vi "DescribeTextField.vi"(0 "XRef":T15, 1 "ID":T3, 2 "State In":T14) -> (14 "Text Field Info":T2, 15 "Fatal Error Out":T1)   [LabVIEW 2022 SP3, in "Flex Block.xnode"]
uses:
  Flex Block.xnode
  <vilib>/XNodeSupport/XNodeXNodeRef.ctl
  <vilib>/XNodeSupport/XNodeString.ctl
  State.ctl
  <vilib>/XNodeSupport/XNodeTextFieldInfo.ctl
  <vilib>/XNodeSupport/XNodeRect32.ctl
  <vilib>/XNodeSupport/XNodeInt.ctl
  <vilib>/XNodeSupport/XNodeJustification.ctl
  <vilib>/XNodeSupport/XNodeHorizontal.ctl
  <vilib>/XNodeSupport/XNodeVertical.ctl
  <vilib>/XNodeSupport/XNodeColor.ctl
  <vilib>/XNodeSupport/XNodeFont.ctl
  <vilib>/XNodeSupport/XNodeUserFont.ctl
  <vilib>/XNodeSupport/XNodeUInt.ctl
  <vilib>/XNodeSupport/XNodeBool.ctl
  <vilib>/XNodeSupport/XNodeErrorCluster.ctl
  <vilib>/XNodeSupport/NI_XNodeSupport.lvlib
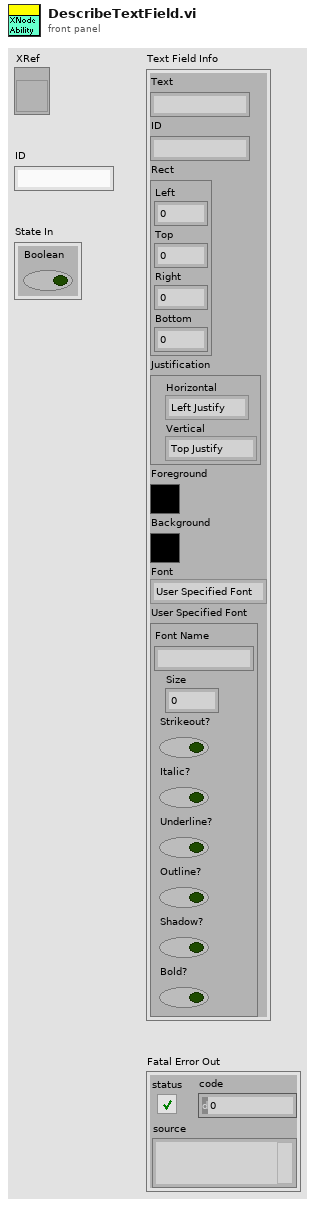
[diagram p1: front panel]
types:
  T1 = typedef "NI_XNodeSupport.lvlib/XNodeErrorCluster.ctl" = errorcluster
  T2 = typedef "NI_XNodeSupport.lvlib/XNodeTextFieldInfo.ctl" = cluster{"Text":T3, "ID":T3, "Rect":T4, "Justification":T6, "Foreground":T9, "Background":T9, "Font":T10, "User Specified Font":T11}
  T3 = typedef "NI_XNodeSupport.lvlib/XNodeString.ctl" = string
  T4 = typedef "NI_XNodeSupport.lvlib/XNodeRect32.ctl" = cluster{"Left":T5, "Top":T5, "Right":T5, "Bottom":T5}
  T5 = typedef "NI_XNodeSupport.lvlib/XNodeInt.ctl" = i32
  T6 = typedef "NI_XNodeSupport.lvlib/XNodeJustification.ctl" = cluster{"Horizontal":T7, "Vertical":T8}
  T7 = typedef "NI_XNodeSupport.lvlib/XNodeHorizontal.ctl" = enum32{"Left Justify", "Right Justify", "CenterJustify"}
  T8 = typedef "NI_XNodeSupport.lvlib/XNodeVertical.ctl" = enum32{"Top Justify", "Bottom Justify", "CenterJustify"}
  T9 = typedef "NI_XNodeSupport.lvlib/XNodeColor.ctl" = u32
  T10 = typedef "NI_XNodeSupport.lvlib/XNodeFont.ctl" = enum32{"User Specified Font", "Application Font", "System Font", "Dialog Font"}
  T11 = typedef "NI_XNodeSupport.lvlib/XNodeUserFont.ctl" = cluster{"Font Name":T3, "Size":T12, "Strikeout?":T13, "Italic?":T13, "Underline?":T13, "Outline?":T13, "Shadow?":T13, "Bold?":T13}
  T12 = typedef "NI_XNodeSupport.lvlib/XNodeUInt.ctl" = u32
  T13 = typedef "NI_XNodeSupport.lvlib/XNodeBool.ctl" = bool
  T14 = typedef "Flex Block.xnode/State.ctl" = cluster{"Boolean":bool}
  T15 = typedef "NI_XNodeSupport.lvlib/XNodeXNodeRef.ctl" = refnum<vi>
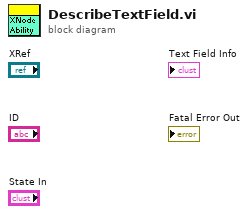
[diagram p0: block diagram]
diagram:
